vi "Read configuration.vi"(8 "error in":errorcluster, 11 "My Awesome Control Modules editor node in":refnum<class "My Awesome Control Modules editor node.lvclass">) -> (0 "error out":errorcluster, 2 "configuration":refnum<class "NISE_CEF_serializable configuration.lvclass">, 3 "My Awesome Control Modules editor node out":refnum<class "My Awesome Control Modules editor node.lvclass">)   [LabVIEW 2013, in "My Awesome Control Modules editor node.lvclass"]
uses:
  My Awesome Control Modules editor node.lvclass
  <vilib>/NI/Configuration Framework/serializable configuration/NISE_CEF_serializable configuration.lvclass
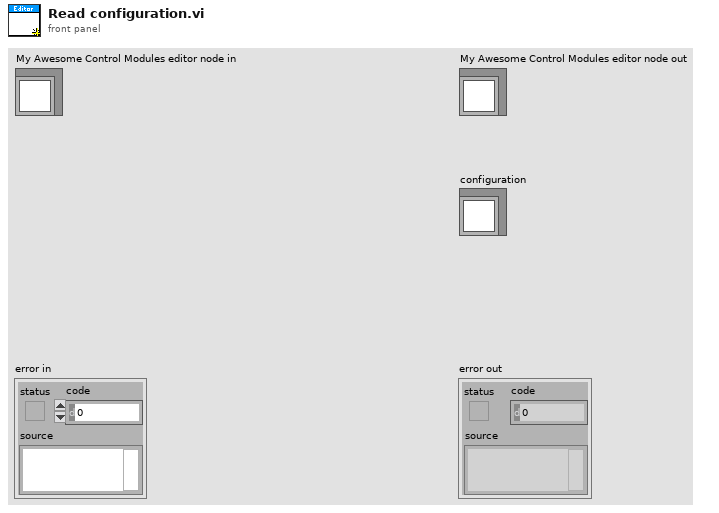
[diagram p1: front panel]
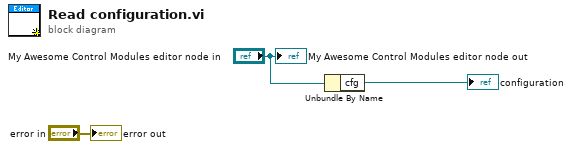
[diagram p0: block diagram]
diagram:
  n1 = Unbundle By Name("My Awesome Control Modules editor node in") -> ("cfg"=→"configuration":refnum<class "My Awesome Control Modules configuration.lvclass">)
  "error out" <- "error in"
  "My Awesome Control Modules editor node out" <- "My Awesome Control Modules editor node in"
